vi "Configure Power Signals Characteristics.vi"(0 "VISA resource name":refnum<visa-resource-name>, 1 "Cycles Number (1)":i32=1, 2 "Duration Time (1E-6 Second)":dbl=1e-06, 3 "Expected Maximum Voltage (20 V)":dbl=20.0, 5 "Cycle Analysis Type (0: Current Harmonics)":i32(ring) items=["Current Harmonics", "Power Quality"], 7 "Duration Analysis Type (0: Efficiency)":i32(ring) items=["Efficiency", "Modulation", "Off", "On", "Ripple", "Transient"], 9 "Vmax Analysis Type (0: INRush)":i32(ring) items=["Inrush", "Off", "On"], 11 "error in (no error)":errorcluster, 12 "Vsteady Analysis Type (0: Off)":i32(ring) items=["Off", "On", "Transient"], 13 "Expected Steady Voltage (20 V)":dbl=20.0) -> (4 "VISA resource name out":refnum<visa-resource-name>, 15 "error out":errorcluster)   [LabVIEW 2010, in "Agilent 2000 3000 X-Series.lvlib"]
doc: "Configure the Power Signals settings. This VI is only applicable for Agilent InfiniiVision 4000 X-Series Oscilloscopes."
uses:
  <instrlib>/Agilent 2000 3000 X-Series/Agilent 2000 3000 X-Series.lvlib
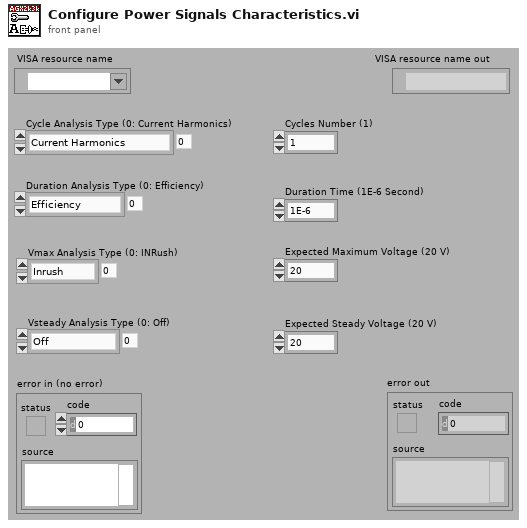
[diagram p1: front panel]
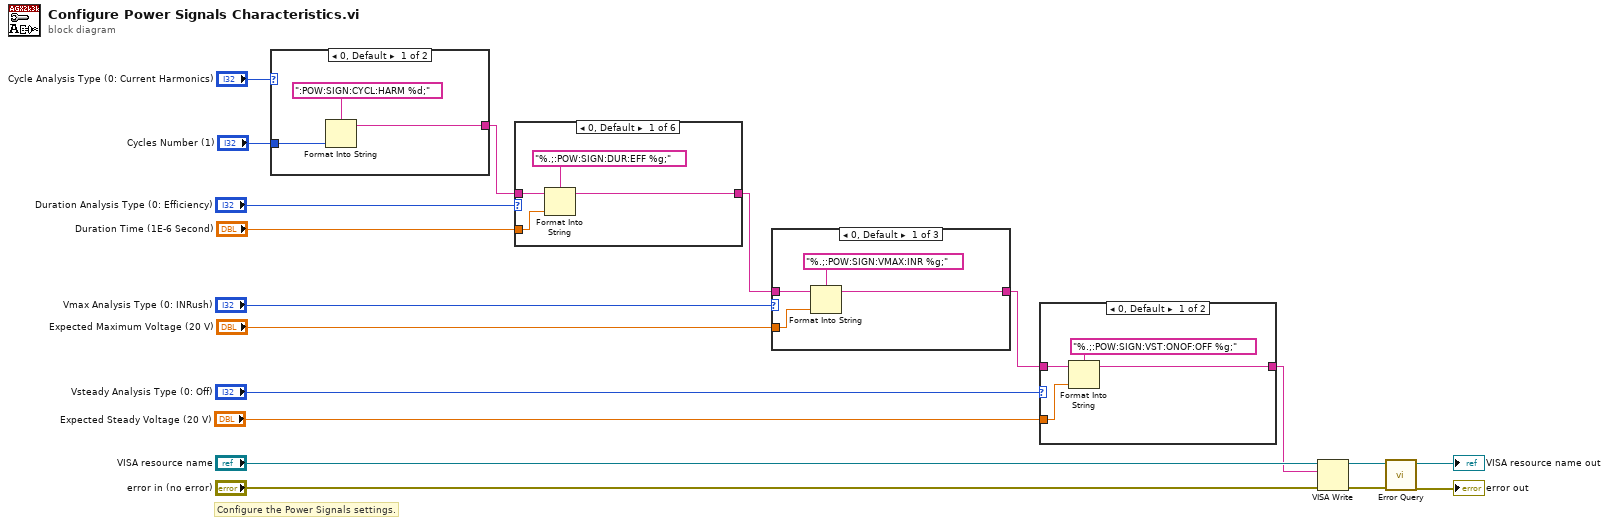
[diagram p0: block diagram]
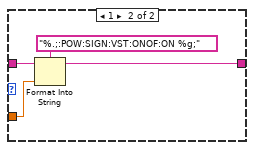
[diagram p2: hidden frame]
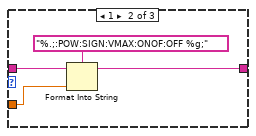
[diagram p3: hidden frame]
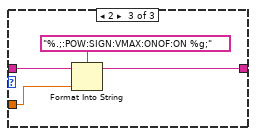
[diagram p4: hidden frame]
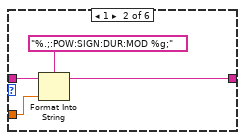
[diagram p5: hidden frame]
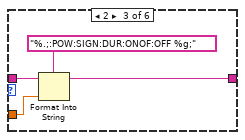
[diagram p6: hidden frame]
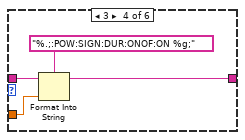
[diagram p7: hidden frame]
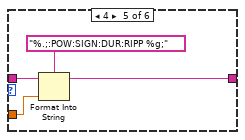
[diagram p8: hidden frame]
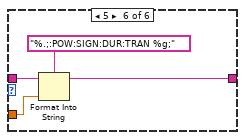
[diagram p9: hidden frame]
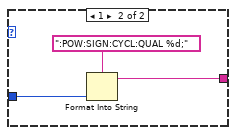
[diagram p10: hidden frame]
diagram:
  # "Configure the Power Signals settings."
  n1 = case shown="0, Default" "Cycle Analysis Type (0: Current Harmonics)" {
    tunnel: "Cycles Number (1)" -> [w19 w23]
    tunnel: [w20 w22] -> w9
    frame 0, Default {
      n2 = Format Into String(format string=":POW:SIGN:CYCL:HARM %d;", w19) -> (resulting string=w20:string)  [unwired: 2 in, 1 out]
    }
    frame 1 {
      n3 = Format Into String(format string=":POW:SIGN:CYCL:QUAL %d;", w23) -> (resulting string=w22:string)  [unwired: 2 in, 1 out]
    }
  }
  n4 = case shown="0, Default" "Duration Analysis Type (0: Efficiency)" {
    tunnel: w9 -> [w27 w32 w36 w40 w44 w48]
    tunnel: [w26 w30 w34 w38 w42 w46] -> w3
    tunnel: "Duration Time (1E-6 Second)" -> [w25 w29 w33 w37 w41 w45]
    frame 0, Default {
      n5 = Format Into String(format string="%.;:POW:SIGN:DUR:EFF %g;", initial string=w27, w25) -> (resulting string=w26:string)  [unwired: 1 in, 1 out]
    }
    frame 1 {
      n6 = Format Into String(format string="%.;:POW:SIGN:DUR:MOD %g;", initial string=w32, w29) -> (resulting string=w30:string)  [unwired: 1 in, 1 out]
    }
    frame 2 {
      n7 = Format Into String(format string="%.;:POW:SIGN:DUR:ONOF:OFF %g;", initial string=w36, w33) -> (resulting string=w34:string)  [unwired: 1 in, 1 out]
    }
    frame 3 {
      n8 = Format Into String(format string="%.;:POW:SIGN:DUR:ONOF:ON %g;", initial string=w40, w37) -> (resulting string=w38:string)  [unwired: 1 in, 1 out]
    }
    frame 4 {
      n9 = Format Into String(format string="%.;:POW:SIGN:DUR:RIPP %g;", initial string=w44, w41) -> (resulting string=w42:string)  [unwired: 1 in, 1 out]
    }
    frame 5 {
      n10 = Format Into String(format string="%.;:POW:SIGN:DUR:TRAN %g;", initial string=w48, w45) -> (resulting string=w46:string)  [unwired: 1 in, 1 out]
    }
  }
  n11 = case shown="0, Default" "Vmax Analysis Type (0: INRush)" {
    tunnel: w3 -> [w52 w56 w60]
    tunnel: [w51 w55 w59] -> w5
    tunnel: "Expected Maximum Voltage (20 V)" -> [w49 w53 w57]
    frame 0, Default {
      n12 = Format Into String(format string="%.;:POW:SIGN:VMAX:INR %g;", initial string=w52, w49) -> (resulting string=w51:string)  [unwired: 1 in, 1 out]
    }
    frame 1 {
      n13 = Format Into String(format string="%.;:POW:SIGN:VMAX:ONOF:OFF %g;", initial string=w56, w53) -> (resulting string=w55:string)  [unwired: 1 in, 1 out]
    }
    frame 2 {
      n14 = Format Into String(format string="%.;:POW:SIGN:VMAX:ONOF:ON %g;", initial string=w60, w57) -> (resulting string=w59:string)  [unwired: 1 in, 1 out]
    }
  }
  n15 = case shown="0, Default" "Vsteady Analysis Type (0: Off)" {
    tunnel: w5 -> [w63 w67]
    tunnel: [w62 w66] -> w4
    tunnel: "Expected Steady Voltage (20 V)" -> [w61 w65]
    frame 0, Default {
      n16 = Format Into String(format string="%.;:POW:SIGN:VST:ONOF:OFF %g;", initial string=w63, w61) -> (resulting string=w62:string)  [unwired: 1 in, 1 out]
    }
    frame 1 {
      n17 = Format Into String(format string="%.;:POW:SIGN:VST:ONOF:ON %g;", initial string=w67, w65) -> (resulting string=w66:string)  [unwired: 1 in, 1 out]
    }
  }
  n18 = VISA Write(VISA resource name="VISA resource name", write buffer=w4, error in (no error)="error in (no error)") -> (VISA resource name out=w16:refnum<visa-resource-name>, error out=w15:errorcluster)  [unwired: 1 out]
  n19 = call <instrlib>:"Error Query.vi"("error in (no error)"=w15, "VISA resource name"=w16) -> ("error out"=→"error out":errorcluster, "VISA resource name out"=→"VISA resource name out":refnum<visa-resource-name>)  [unwired: 8 out]
